vi "Send $PO.vi"(8 "error in (no error)":errorcluster, 11 "LTI ULS Actor in":refnum<class "LTI ULS Actor.lvclass">) -> (0 "error out":errorcluster, 3 "LTI ULS Actor out":refnum<class "LTI ULS Actor.lvclass">)   [LabVIEW 2018, in "LTI ULS Actor.lvlib" / "LTI ULS Actor.lvclass"]
uses:
  LTI ULS Actor.lvclass
  C:/Users/dev/Documents/CODE/LabVIEW/microwaveverify/trunk/MWWL Verification/Sensor Actor/Sensor/Sensor.lvclass
  Sensor Actor/Sensor/Sensor.lvclass
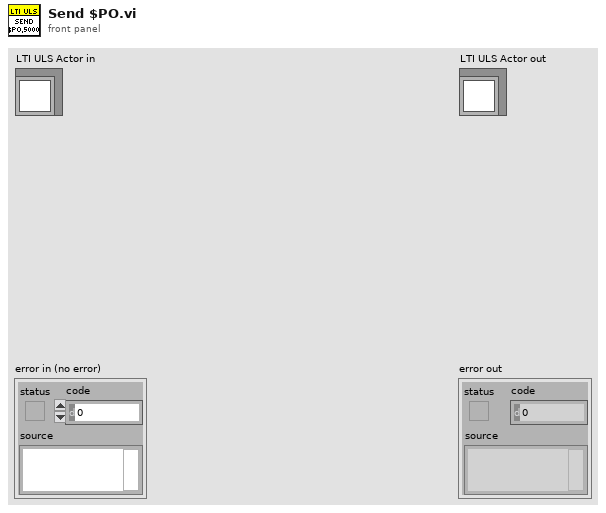
[diagram p1: front panel]
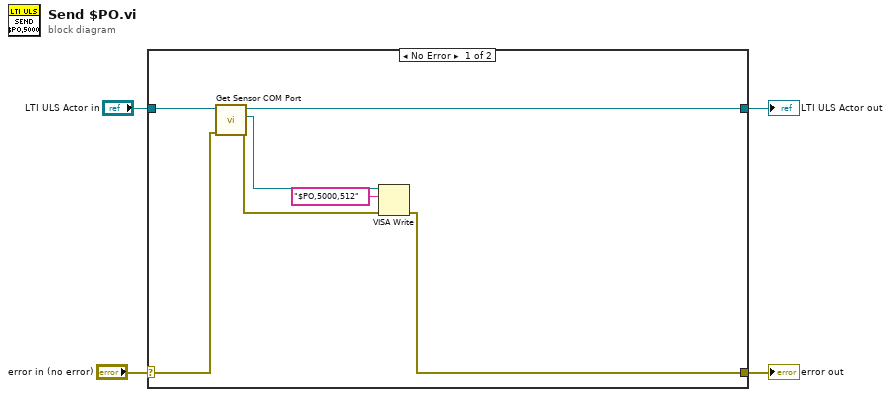
[diagram p0: block diagram]
diagram:
  n1 = case shown="No Error" "error in (no error)" {
    selector: "error in (no error)" -> [w6 w13]
    tunnel: [w5 w13] -> w3
    tunnel: [w10 w12] -> w1
    tunnel: "LTI ULS Actor in" -> [w11 w12]
    frame No Error {
      n2 = call "Get Sensor COM Port.vi"("error in (no error)"=w6, "Sensor in"=w11) -> ("error out"=w7:errorcluster, "COM Port"=w9:refnum<visa-resource-name>, "Sensor out"=w10:refnum<class "LTI ULS Actor.lvclass">)  [unwired: 7 in]
      n3 = VISA Write(VISA resource name=w9, write buffer="$PO,5000,512", error in (no error)=w7) -> (error out=w5:errorcluster)  [unwired: 2 out]
    }
    frame Error {
    }
  }
  "error out" <- w3
  "LTI ULS Actor out" <- w1
